vi "AMI135Monitor.vi"() -> ()   [LabVIEW 2016]
uses:
  Instrument_Setup.vi
  Global/Global Variables/Data_Display_global.vi
panel:
  in  "error in 2":T1
  out "Helium (%)":dbl
  out "error out":T1
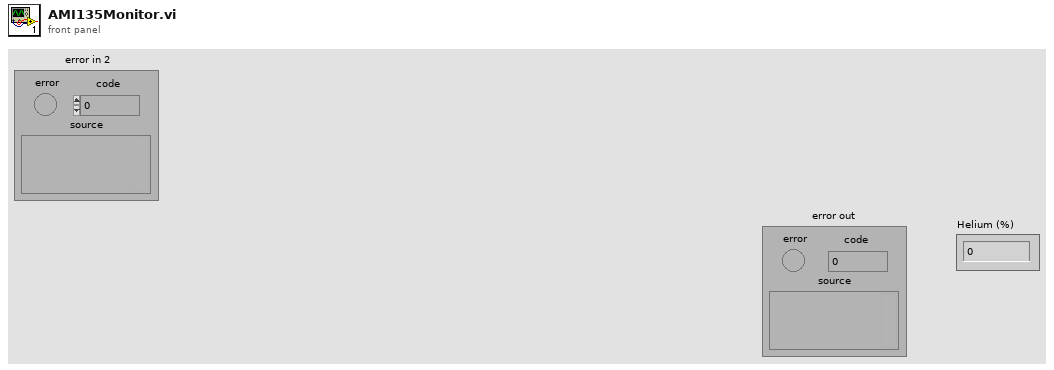
[diagram p1: front panel]
types:
  T1 = cluster{"error":bool, "code":i32, "source":string}
  T2 = cluster{"Sensor Length (cm)":sgl, "Hi Setpoint (cm)":sgl, "Lo Setpoint (cm)":sgl, "Sampling Interval (min)":sgl}
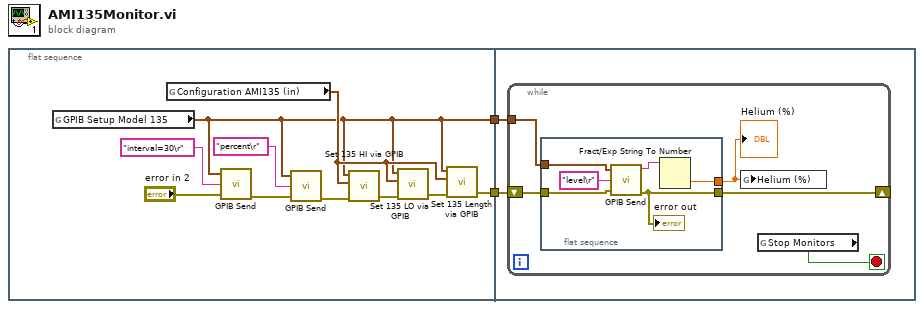
[diagram p0: block diagram]
diagram:
  n1 = flat-sequence {
    tunnel: [w3] -> w2
    tunnel: [w7] -> w1
    tunnel: w2 -> [w14]
    tunnel: w1 -> [w13]
    frame #0 {
      n2 = global read "Instrument_Setup.vi" "GPIB Setup Model 135"() -> (w7:cluster{"GPIB address":i16, "GPIB bus":i16})
      n3 = global read "Instrument_Setup.vi" "Configuration AMI135 (in)"() -> (w8:T2)
      n4 = call "GPIB Send.vi"("GPIB Setup"=w7, "Input command"="interval=30\r", "error in"="error in 2") -> ("error out"=w9:T1)  [unwired: 3 out]
      n5 = call "GPIB Send.vi"("GPIB Setup"=w7, "Input command"="percent\r", "error in"=w9) -> ("error out"=w6:T1)  [unwired: 3 out]
      n6 = call "Set 135 HI via GPIB.vi"("error in"=w6, "Configuration (in)"=w8, "GPIB Setup"=w7) -> ("error out"=w5:T1)  [unwired: 1 in, 2 out]
      n7 = call "Set 135 LO via GPIB.vi"("error in"=w5, "Configuration (in)"=w8, "GPIB Setup"=w7) -> ("error out"=w4:T1)  [unwired: 1 in, 2 out]
      n8 = call "Set 135 Length via GPIB.vi"("error in"=w4, "Configuration (in)"=w8, "GPIB Setup"=w7) -> ("error out"=w3:T1)  [unwired: 1 in, 2 out]
    }
    frame #1 {
      n9 = while {
        shift-right: [w18] -> _
        shift-left: w14 -> [w15]
        tunnel: w13 -> [w16]
        stop <- w17 stop-if-true
        n10 = flat-sequence {
          tunnel: [w23] -> w19
          tunnel: [w22] -> w18
          tunnel: w16 -> [w21]
          tunnel: w15 -> [w20]
          frame #0 {
            n11 = call "GPIB Send.vi"("GPIB Setup"=w21, "Input command"="level\r", "error in"=w20) -> ("Return string"=w24:string, "error out"=w22:T1)  [unwired: 2 out]
            "error out" <- w22
            n12 = Fract/Exp String To Number(string=w24) -> (number=w23:dbl)  [unwired: 3 in, 1 out]
          }
        }
        n13 = global write "Data_Display_global.vi" "Helium (%)"(w19) -> ()
        n14 = global read "Data_Display_global.vi" "Stop Monitors"() -> (w17:bool)
        "Helium (%)" <- w19
      }
    }
  }
